vi "Lab Panel V4.82.vi"() -> ()   [LabVIEW 2013] (continued)
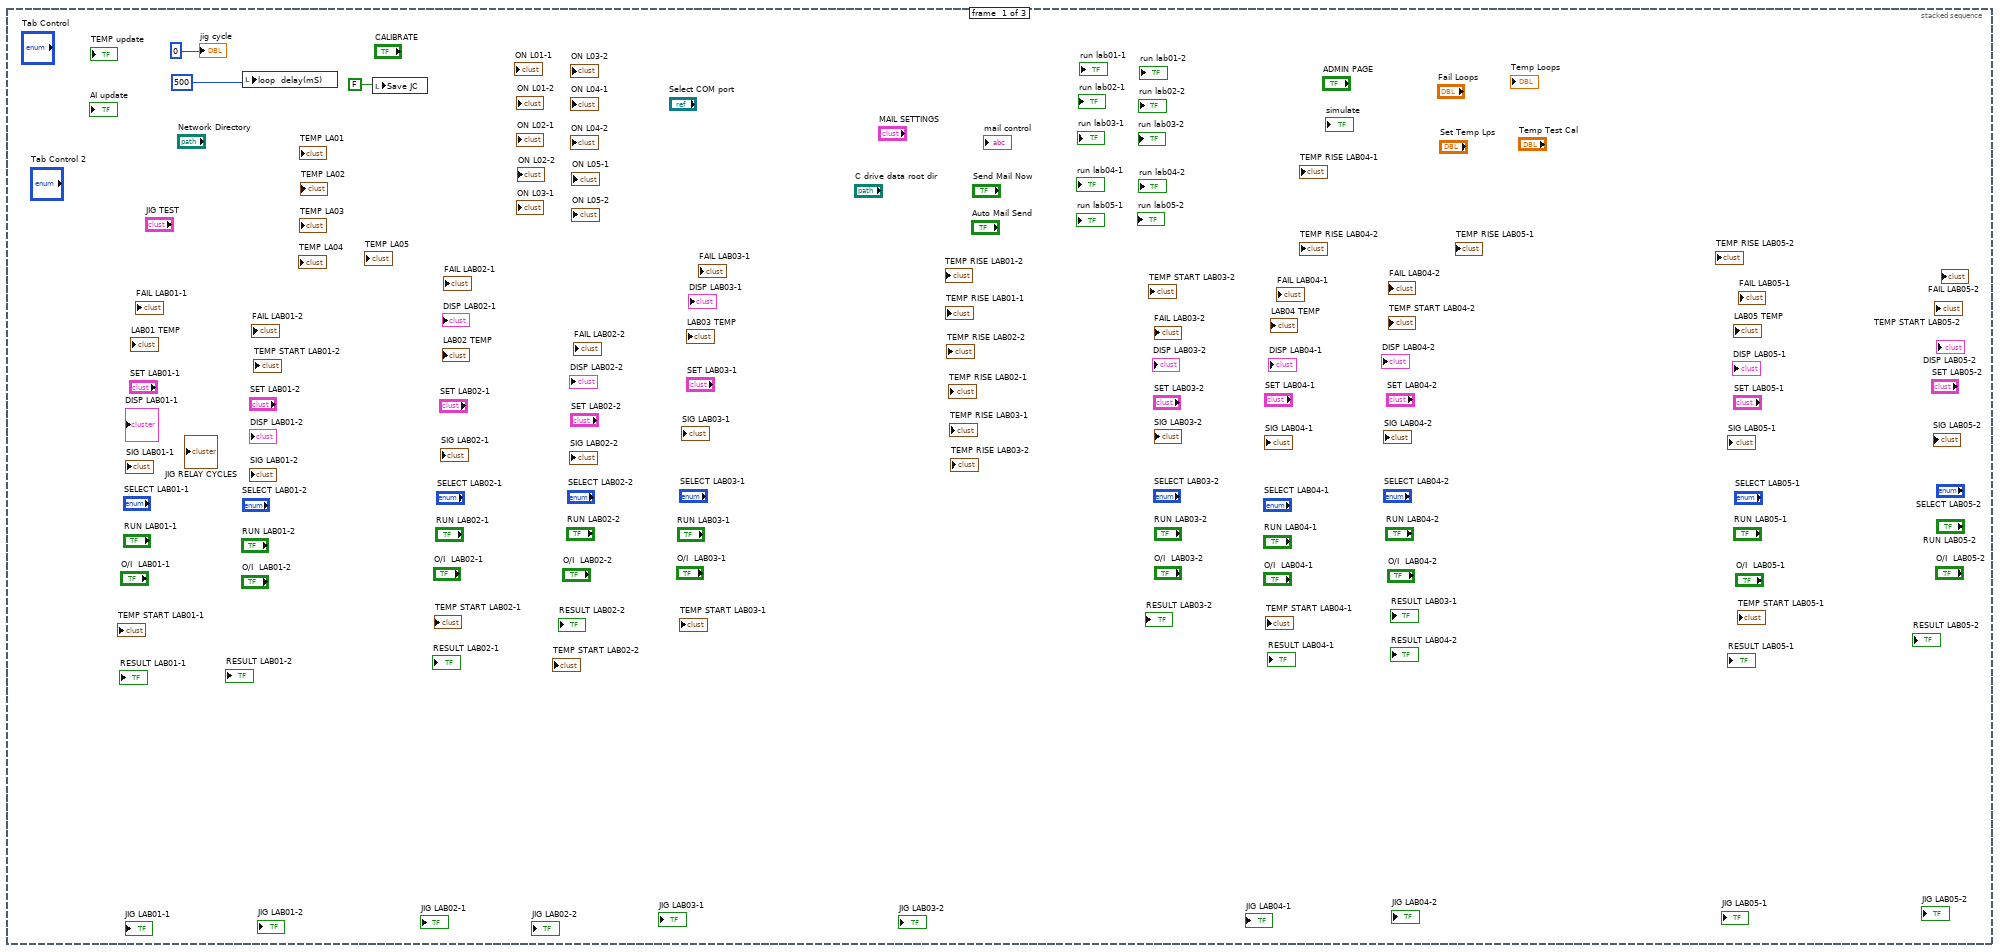
[diagram p2: hidden frame]
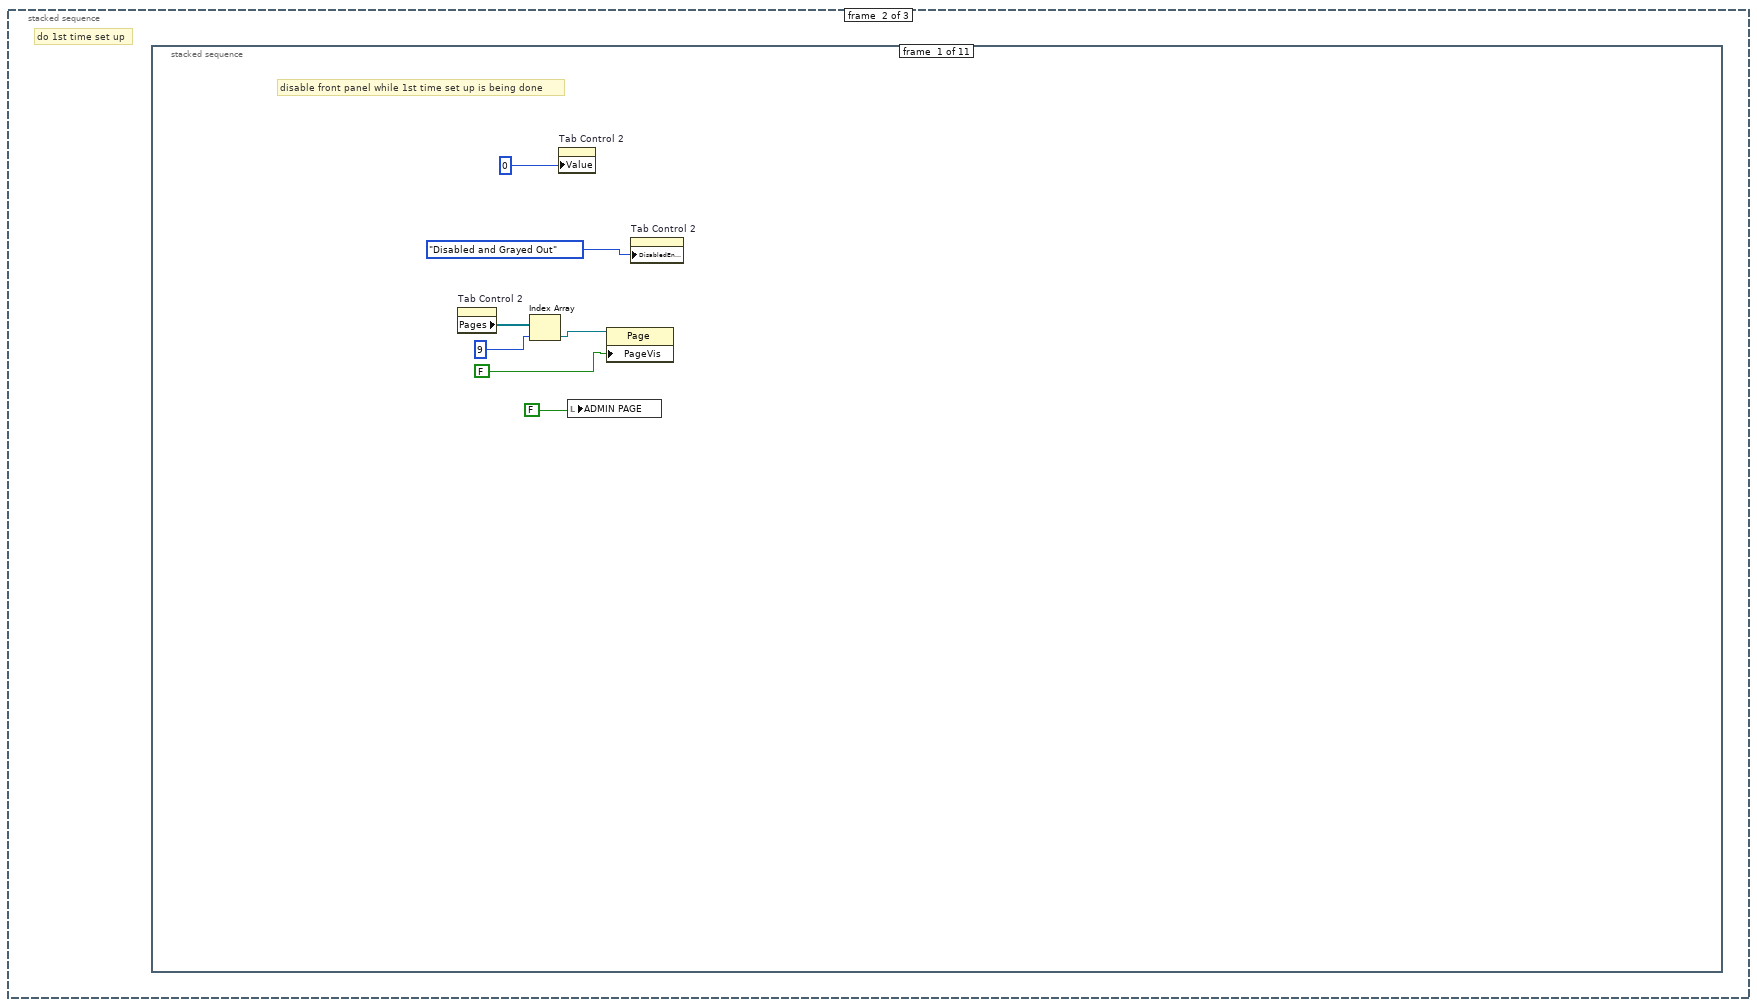
[diagram p3: hidden frame]
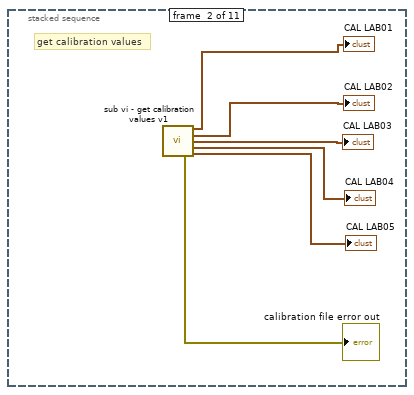
[diagram p4: hidden frame]
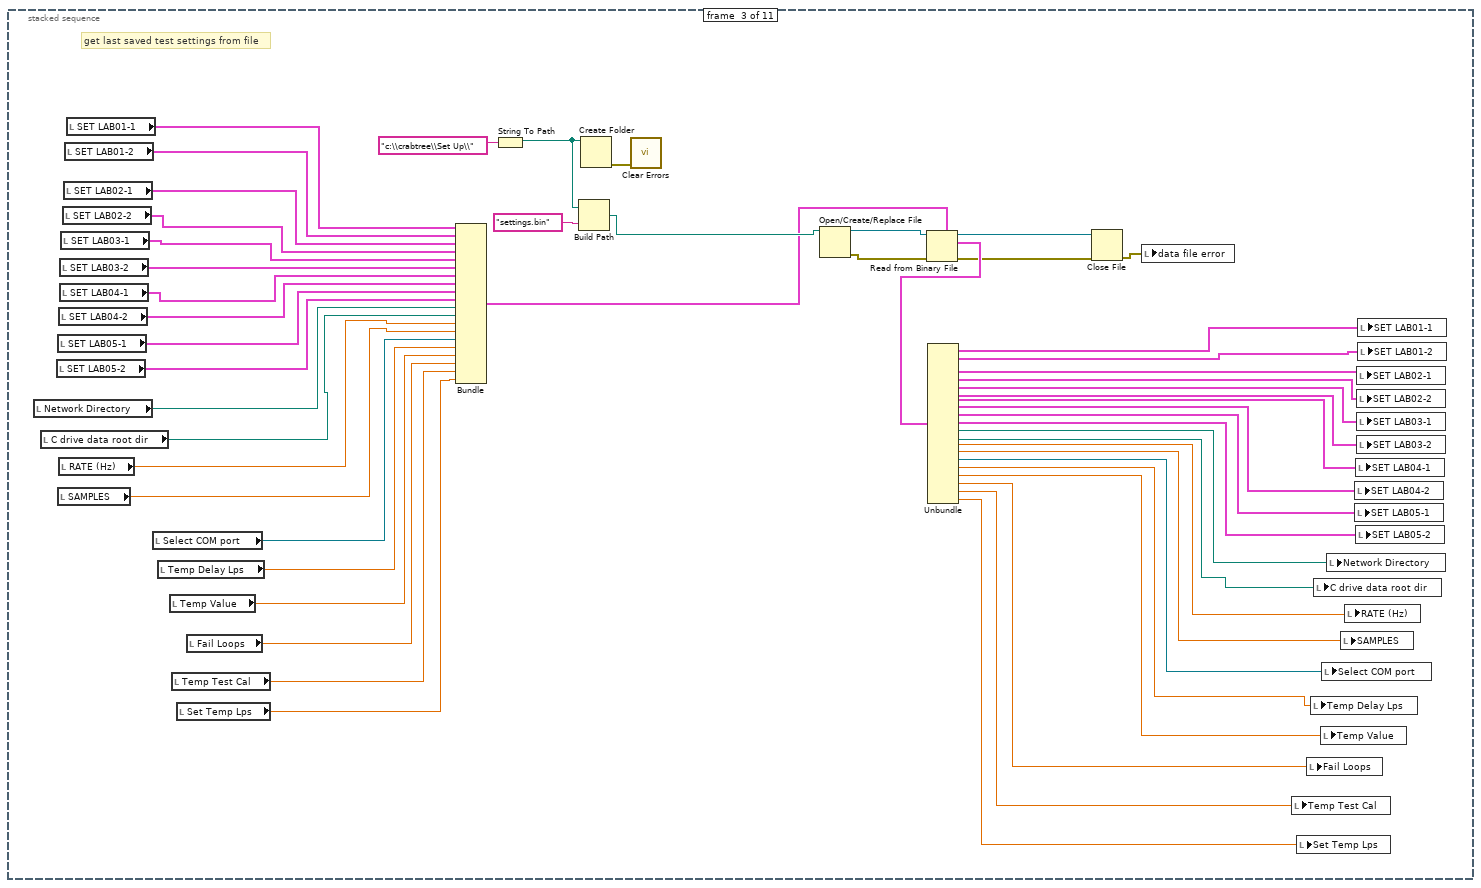
[diagram p5: hidden frame]
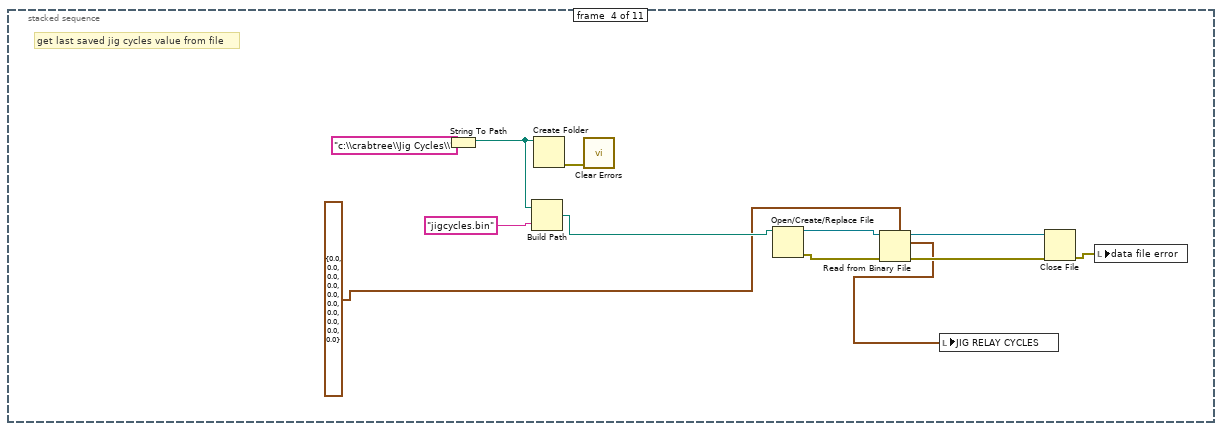
[diagram p6: hidden frame]
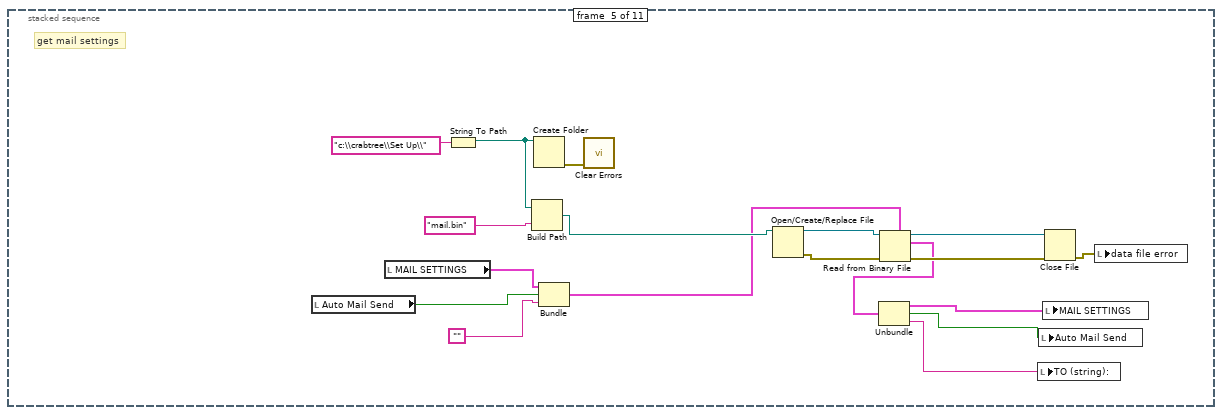
[diagram p7: hidden frame]
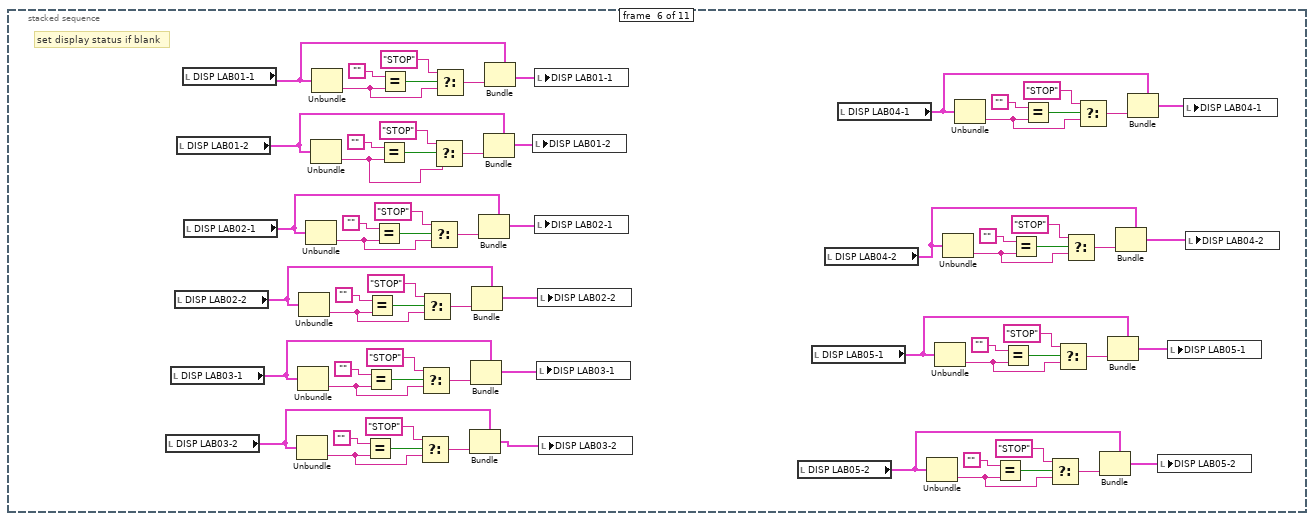
[diagram p8: hidden frame]
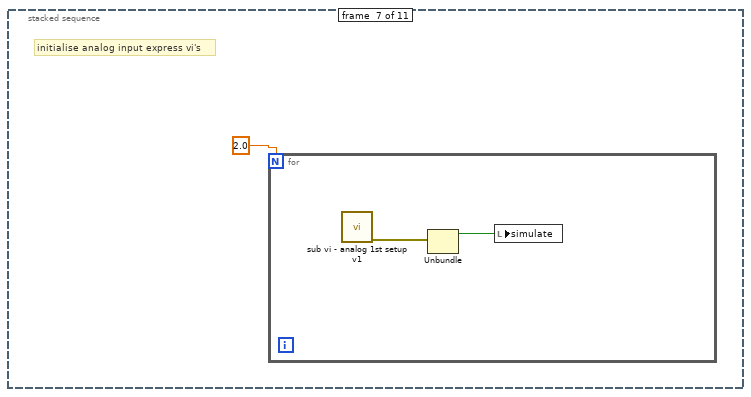
[diagram p9: hidden frame]
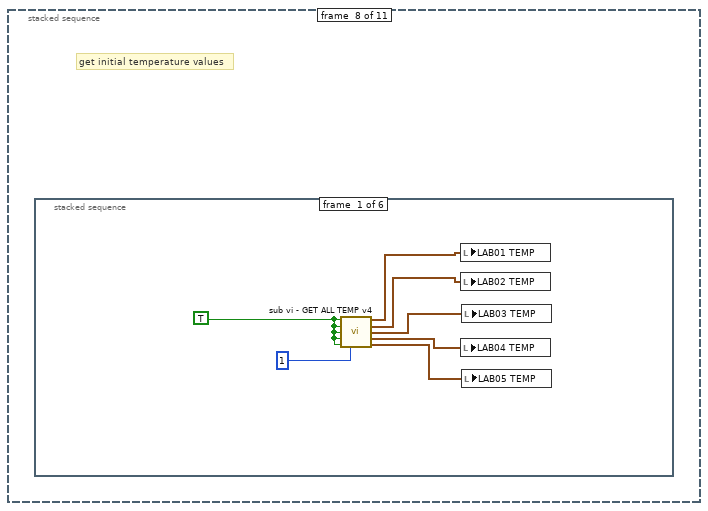
[diagram p10: hidden frame]
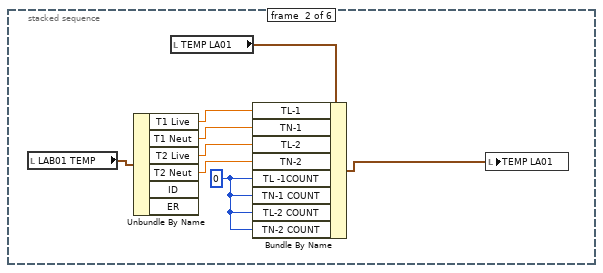
[diagram p11: hidden frame]
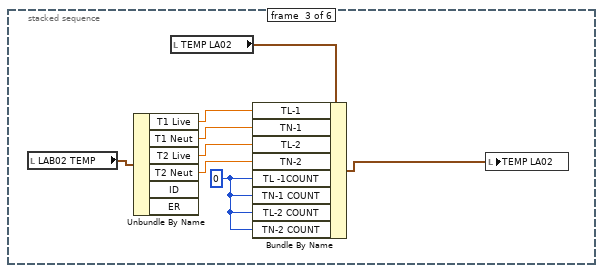
[diagram p12: hidden frame]
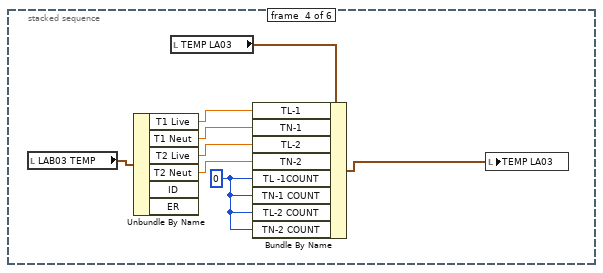
[diagram p13: hidden frame]
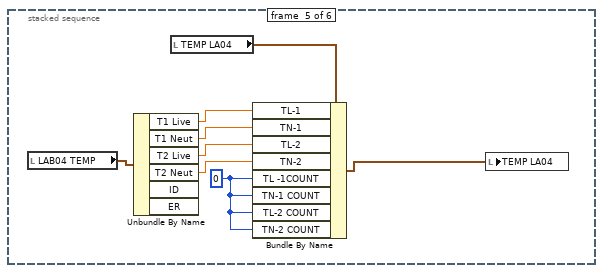
[diagram p14: hidden frame]
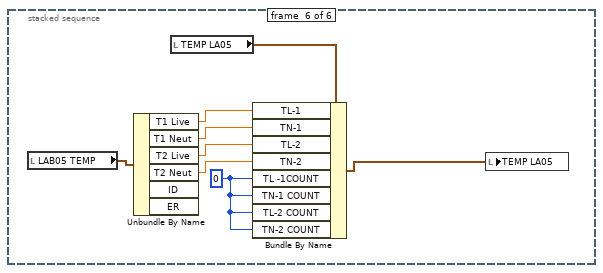
[diagram p15: hidden frame]
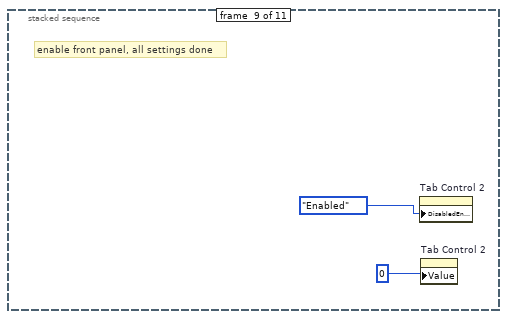
[diagram p16: hidden frame]
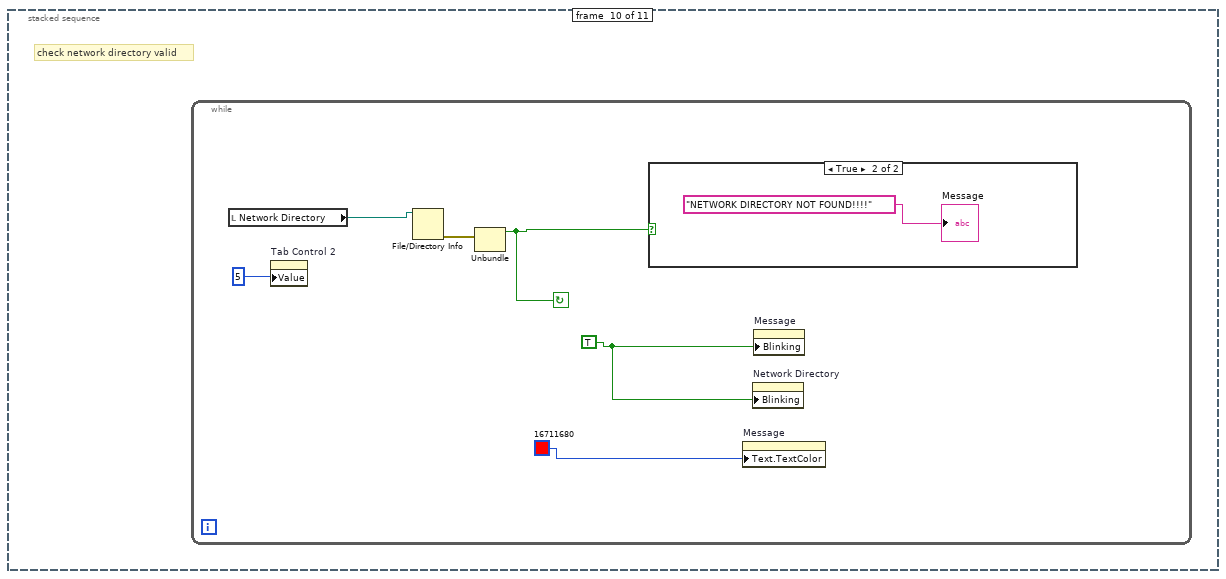
[diagram p17: hidden frame]
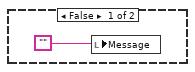
[diagram p18: hidden frame]
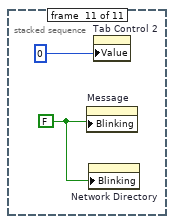
[diagram p19: hidden frame]
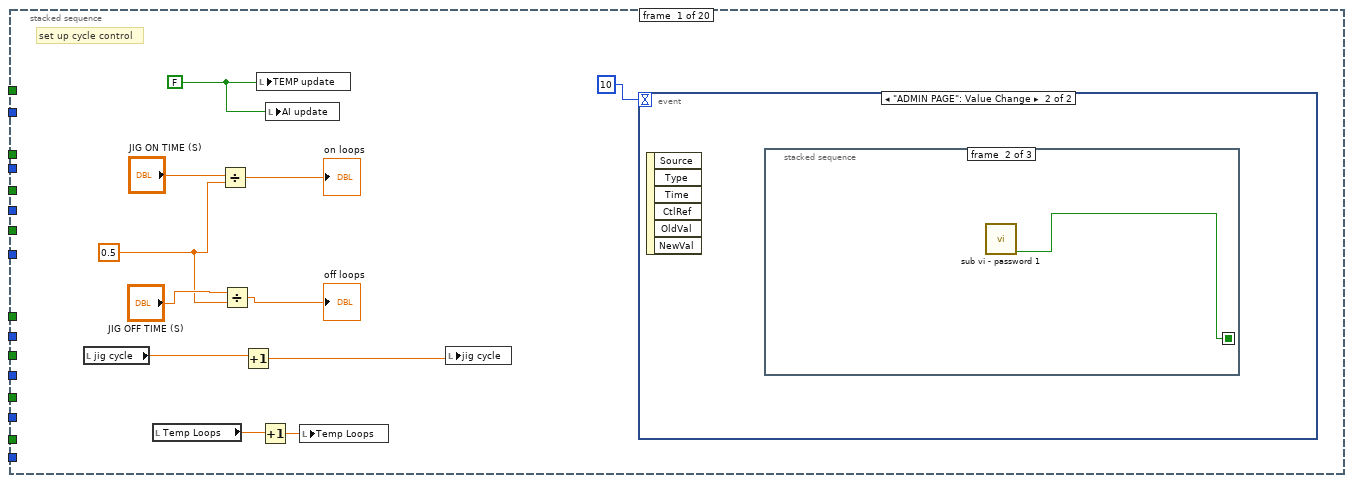
[diagram p20: hidden frame]
                            n2643 = Greater?(x=w4490, y=w4493) -> (0:w4492:bool)
                            n2644 = case shown="True" w4492 {
                              tunnel: [w4494 0] -> w4491
                              tunnel: w4490 -> [w4494 _]
                              tunnel: w4489 -> [_ w4495]
                              frame False {
                              }
                              frame True {
                                n2645 = Concatenate Strings("LA01-1 ", w4495) -> (w4498:string)
                                n2646 = One Button Dialog(message=w4498) -> ()  [unwired: 1 in, 1 out]
                              }
                            }
                          }
                          frame #1 {
                            n2647 = Greater?(x=w4499, y=w4503) -> (0:w4502:bool)
                            n2648 = case shown="True" w4502 {
                              tunnel: [w4504 0] -> w4500
                              tunnel: w4499 -> [w4504 _]
                              tunnel: w4501 -> [_ w4505]
                              frame False {
                              }
                              frame True {
                                n2649 = Concatenate Strings("LA01-2 ", w4505) -> (w4508:string)
                                n2650 = One Button Dialog(message=w4508) -> ()  [unwired: 1 in, 1 out]
                              }
                            }
                          }
                          frame #2 {
                            n2651 = Greater?(x=w4509, y=w4513) -> (0:w4512:bool)
                            n2652 = case shown="True" w4512 {
                              tunnel: [w4514 0] -> w4510
                              tunnel: w4509 -> [w4514 _]
                              tunnel: w4511 -> [_ w4515]
                              frame False {
                              }
                              frame True {
                                n2653 = Concatenate Strings("LA02-1 ", w4515) -> (w4518:string)
                                n2654 = One Button Dialog(message=w4518) -> ()  [unwired: 1 in, 1 out]
                              }
                            }
                          }
                          frame #3 {
                            n2655 = Greater?(x=w4520, y=w4523) -> (0:w4522:bool)
                            n2656 = case shown="True" w4522 {
                              tunnel: [w4524 0] -> w4519
                              tunnel: w4520 -> [w4524 _]
                              tunnel: w4521 -> [_ w4525]
                              frame False {
                              }
                              frame True {
                                n2657 = Concatenate Strings("LA02-2 ", w4525) -> (w4528:string)
                                n2658 = One Button Dialog(message=w4528) -> ()  [unwired: 1 in, 1 out]
                              }
                            }
                          }
                          frame #4 {
                            n2659 = Greater?(x=w4530, y=w4533) -> (0:w4532:bool)
                            n2660 = case shown="True" w4532 {
                              tunnel: [w4534 0] -> w4529
                              tunnel: w4530 -> [w4534 _]
                              tunnel: w4531 -> [_ w4535]
                              frame False {
                              }
                              frame True {
                                n2661 = Concatenate Strings("LA03-1 ", w4535) -> (w4538:string)
                                n2662 = One Button Dialog(message=w4538) -> ()  [unwired: 1 in, 1 out]
                              }
                            }
                          }
                          frame #5 {
                            n2663 = Greater?(x=w4539, y=w4543) -> (0:w4542:bool)
                            n2664 = case shown="True" w4542 {
                              tunnel: [w4544 0] -> w4540
                              tunnel: w4539 -> [w4544 _]
                              tunnel: w4541 -> [_ w4545]
                              frame False {
                              }
                              frame True {
                                n2665 = Concatenate Strings("LA03-2 ", w4545) -> (w4548:string)
                                n2666 = One Button Dialog(message=w4548) -> ()  [unwired: 1 in, 1 out]
                              }
                            }
                          }
                          frame #6 {
                            n2667 = Greater?(x=w4550, y=w4553) -> (0:w4552:bool)
                            n2668 = case shown="True" w4552 {
                              tunnel: [w4554 0] -> w4549
                              tunnel: w4550 -> [w4554 _]
                              tunnel: w4551 -> [_ w4555]
                              frame False {
                              }
                              frame True {
                                n2669 = Concatenate Strings("LA04-1 ", w4555) -> (w4558:string)
                                n2670 = One Button Dialog(message=w4558) -> ()  [unwired: 1 in, 1 out]
                              }
                            }
                          }
                          frame #7 {
                            n2671 = Greater?(x=w4560, y=w4563) -> (0:w4562:bool)
                            n2672 = case shown="True" w4562 {
                              tunnel: [w4564 0] -> w4559
                              tunnel: w4560 -> [w4564 _]
                              tunnel: w4561 -> [_ w4565]
                              frame False {
                              }
                              frame True {
                                n2673 = Concatenate Strings("LA04-2 ", w4565) -> (w4568:string)
                                n2674 = One Button Dialog(message=w4568) -> ()  [unwired: 1 in, 1 out]
                              }
                            }
                          }
                          frame #8 {
                            n2675 = Greater?(x=w4570, y=w4573) -> (0:w4572:bool)
                            n2676 = case shown="True" w4572 {
                              tunnel: [w4574 0] -> w4569
                              tunnel: w4570 -> [w4574 _]
                              tunnel: w4571 -> [_ w4575]
                              frame False {
                              }
                              frame True {
                                n2677 = Concatenate Strings("LA05-1 ", w4575) -> (w4578:string)
                                n2678 = One Button Dialog(message=w4578) -> ()  [unwired: 1 in, 1 out]
                              }
                            }
                          }
                          frame #9 {
                            n2679 = Greater?(x=w4580, y=w4583) -> (0:w4582:bool)
                            n2680 = case shown="True" w4582 {
                              tunnel: [w4584 0] -> w4579
                              tunnel: w4580 -> [w4584 _]
                              tunnel: w4581 -> [_ w4585]
                              frame False {
                              }
                              frame True {
                                n2681 = Concatenate Strings("LA05-2 ", w4585) -> (w4588:string)
                                n2682 = One Button Dialog(message=w4588) -> ()  [unwired: 1 in, 1 out]
                              }
                            }
                          }
                        }
                        n2683 = Bundle By Name(cluster=w4487, "LAB01-1"=w4485, "LAB01-2"=w4483, "LAB02-1"=w4480, "LAB02-2"=w4477, "LAB03-1"=w4475, "LAB03-2"=w4474, "LAB04-1"=w4471, "LAB04-2"=w4469, "LAB05-1"=w4467, "LAB05-2"=w4465) -> (w4486:T10)
                        n2684 = local write "JIG RELAY CYCLES"(w4486) -> ()
                      }
                    }
                  }
                }
              }
            }
          }
          frame #19 {
            # "get temperature values"
            n2685 = local read "simulate"() -> (w4593:bool)
            n2686 = local read "Temp Test Cal"() -> (w4590:dbl)
            n2687 = stacked-sequence {
              tunnel: w4593 -> [_ w4631 w4660 w4684 w4708 w4732]
              tunnel: T8 {"1  (A) cal"=1.0, "1 (V) cal"=1.0, "1 (PF) cal"=1.0, "1 (TL) cal"=1.0, "1 (TN) cal"=1.0, "2 (A) cal"=1.0, "2 (V) cal"=1.0, "2 (PF) cal"=1.0, "2 (TL) cal"=1.0, "2 (TN) cal"=1.0} ("CAL LAB01") -> [_ w4630 w4659 w4683 w4707 w4731]
              tunnel: w4591 -> [_ w4628 _ _ _ _]
              tunnel: w4590 -> [_ w4626 _ _ _ _]
              tunnel: w4589 -> [_ _ _ _ _ _]
              frame #0 {
                n2688 = local read "Select COM port"() -> (w4602:refnum<visa-resource-name>)
                "COM port" <- w4602
                n2689 = local read "Set Temp Lps"() -> (w4594:dbl)
                n2690 = local read "jig cycle"() -> (w4603:dbl)
                n2691 = local read "on loops"() -> (w4605:dbl)
                n2692 = local read "Temp Loops"() -> (w4598:dbl)
                n2693 = global write "Global 1.vi" "tmp dly lps"("Temp Delay Lps") -> ()
                n2694 = global write "Global 1.vi" "dly value"("Temp Value") -> ()
                n2695 = Add(x=w4605, y=3) -> (x+y=w4606:dbl)
                n2696 = global write "Global 1.vi" "COM port"(w4602) -> ()
                n2697 = Equal?(x=w4603, y=w4606) -> (x = y?=w4597:bool)
                n2698 = Greater Or Equal?(x=w4598, y=w4594) -> (x >= y?=w4596:bool)
                n2699 = And(x=w4597, y=w4596) -> (x .and. y?=w4595:bool)
                n2700 = local read "simulate"() -> (w4599:bool)
                n2701 = case shown="True" w4595 {
                  tunnel: w4599 -> [_ w4611]
                  frame False {
                  }
                  frame True {
                    n2702 = case shown="False" w4611 {
                      tunnel: [w4619 w4623] -> w4613
                      tunnel: [w4618 w4623] -> w4612
                      tunnel: [w4617 w4623] -> w4610
                      tunnel: [w4616 w4623] -> w4609
                      tunnel: [w4615 w4623] -> w4608
                      frame False {
                        w4621 = TRUE
                        w4622 = TRUE
                        n2703 = call "sub vi - GET ALL TEMP v4.vi"("LA01-EN"=w4622, "LA02-EN"=w4622, "LA03-EN"=w4622, "LA04-EN"=w4621, "LA05-EN"=w4621, "Gen Cal Value"=1.0) -> ("LA01 TEMP"=w4615:T23, "LA02 TEMP"=w4616:T23, "LA03 TEMP"=w4617:T23, "LA04 TEMP"=w4619:T23, "LA05 TEMP"=w4618:T23)  [unwired: 4 in, 1 out]
                      }
                      frame True {
                        w4623 = T14 {"T1 Live"=21.0, "T1 Neut"=22.0, "T2 Live"=23.0, "T2 Neut"=24.0, "ID"=6.0, "ER"=10.0} ("LAB01 TEMP")
                      }
                    }
                    n2704 = local write "Temp Loops"(0) -> ()
                    n2705 = local write "TEMP update"(TRUE) -> ()
                    n2706 = local write "LAB03 TEMP"(w4610) -> ()
                    n2707 = local write "LAB02 TEMP"(w4609) -> ()
                    n2708 = local write "LAB04 TEMP"(w4613) -> ()
                    n2709 = local write "LAB05 TEMP"(w4612) -> ()
                    n2710 = local write "LAB01 TEMP"(w4608) -> ()
                  }
                }
              }
              frame #1 {
                n2711 = case shown="False" w4631 {
                  tunnel: [w4657 w4658] -> w4649
                  tunnel: w4630 -> [_ w4658]
                  frame False {
                    n2712 = local read "CAL LAB01"() -> (w4657:T8)
                  }
                  frame True {
                  }
                }
                n2713 = local read "LAB01 TEMP"() -> (w4637:T14)
                n2714 = local read "TEMP LA01"() -> (w4638:T11)
                n2715 = call "sub vi - temperature delay v2.vi"("temp values IN"=w4638, "temp signals"=w4637) -> ("T2-N"=w4633:dbl, "T2-L"=w4634:dbl, "T1-N"=w4635:dbl, "T1-L"=w4636:dbl, "temp values OUT"=w4632:T43)  [unwired: 5 in]
                n2716 = Unbundle By Name(w4649) -> ("1 (TL) cal"=w4642:dbl, "1 (TN) cal"=w4641:dbl, "2 (TL) cal"=w4640:dbl, "2 (TN) cal"=w4639:dbl)  [unwired: 6 out]
                n2717 = local write "TEMP LA01"(w4632) -> ()
                n2718 = Multiply(x=w4636, y=w4642) -> (x*y=w4629:dbl)
                n2719 = Multiply(x=w4635, y=w4641) -> (x*y=w4625:dbl)
                n2720 = Multiply(x=w4634, y=w4640) -> (x*y=w4644:dbl)
                n2721 = Multiply(x=w4633, y=w4639) -> (x*y=w4643:dbl)
                n2722 = case shown="True" w4628 {
                  tunnel: w4629 -> [w4651 w4656]
                  tunnel: w4626 -> [_ w4654]
                  tunnel: [w4651 w4655] -> w4627
                  tunnel: w4625 -> [w4650 w4653]
                  tunnel: [w4650 w4652] -> w4624
                  frame False {
                  }
                  frame True {
                    n2723 = Multiply(x=w4654, y=w4653) -> (x*y=w4652:dbl)
                    n2724 = Multiply(x=w4654, y=w4656) -> (x*y=w4655:dbl)
                  }
                }
                n2725 = local read "SIG LAB01-2"() -> (w4646:T2)
                n2726 = local read "SIG LAB01-1"() -> (w4648:T2)
                n2727 = Bundle By Name(cluster=w4648, "Tmp Live"=w4627, "Tmp Neut"=w4624) -> (w4647:T2)
                n2728 = Bundle By Name(cluster=w4646, "Tmp Live"=w4644, "Tmp Neut"=w4643) -> (w4645:T2)
                n2729 = local write "SIG LAB01-1"(w4647) -> ()
                n2730 = local write "SIG LAB01-2"(w4645) -> ()
              }
              frame #2 {
                n2731 = case shown="True" w4660 {
                  tunnel: [w4681 w4682] -> w4680
                  tunnel: w4659 -> [_ w4682]
                  frame False {
                    n2732 = local read "CAL LAB02"() -> (w4681:T9)
                  }
                  frame True {
                  }
                }
                n2733 = local read "LAB02 TEMP"() -> (w4667:T14)
                n2734 = local read "TEMP LA02"() -> (w4666:T11)
                n2735 = call "sub vi - temperature delay v2.vi"("temp values IN"=w4666, "temp signals"=w4667) -> ("T2-N"=w4661:dbl, "T2-L"=w4662:dbl, "T1-N"=w4663:dbl, "T1-L"=w4664:dbl, "temp values OUT"=w4665:T43)  [unwired: 5 in]
                n2736 = Unbundle By Name(w4680) -> ("1 (TL) cal"=w4671:dbl, "1 (TN) cal"=w4670:dbl, "2 (TL) cal"=w4669:dbl, "2 (TN) cal"=w4668:dbl)  [unwired: 6 out]
                n2737 = local write "TEMP LA02"(w4665) -> ()
                n2738 = Multiply(x=w4664, y=w4671) -> (x*y=w4677:dbl)
                n2739 = Multiply(x=w4663, y=w4670) -> (x*y=w4676:dbl)
                n2740 = Multiply(x=w4662, y=w4669) -> (x*y=w4673:dbl)
                n2741 = Multiply(x=w4661, y=w4668) -> (x*y=w4672:dbl)
                n2742 = local read "SIG LAB02-2"() -> (w4675:T2)
                n2743 = local read "SIG LAB02-1"() -> (w4679:T2)
                n2744 = Bundle By Name(cluster=w4679, "Tmp Live"=w4677, "Tmp Neut"=w4676) -> (w4678:T2)
                n2745 = Bundle By Name(cluster=w4675, "Tmp Live"=w4673, "Tmp Neut"=w4672) -> (w4674:T2)
                n2746 = local write "SIG LAB02-1"(w4678) -> ()
                n2747 = local write "SIG LAB02-2"(w4674) -> ()
              }
              frame #3 {
                n2748 = case shown="False" w4684 {
                  tunnel: [w4705 w4706] -> w4704
                  tunnel: w4683 -> [_ w4706]
                  frame False {
                    n2749 = local read "CAL LAB03"() -> (w4705:T8)
                  }
                  frame True {
                  }
                }
                n2750 = local read "TEMP LA03"() -> (w4690:T11)
                n2751 = local read "LAB03 TEMP"() -> (w4691:T14)
                n2752 = call "sub vi - temperature delay v2.vi"("temp values IN"=w4690, "temp signals"=w4691) -> ("T2-N"=w4685:dbl, "T2-L"=w4686:dbl, "T1-N"=w4687:dbl, "T1-L"=w4688:dbl, "temp values OUT"=w4689:T43)  [unwired: 5 in]
                n2753 = Unbundle By Name(w4704) -> ("1 (TL) cal"=w4695:dbl, "1 (TN) cal"=w4694:dbl, "2 (TL) cal"=w4693:dbl, "2 (TN) cal"=w4692:dbl)  [unwired: 6 out]
                n2754 = local write "TEMP LA03"(w4689) -> ()
                n2755 = Multiply(x=w4688, y=w4695) -> (x*y=w4701:dbl)
                n2756 = Multiply(x=w4687, y=w4694) -> (x*y=w4700:dbl)
                n2757 = Multiply(x=w4686, y=w4693) -> (x*y=w4697:dbl)
                n2758 = Multiply(x=w4685, y=w4692) -> (x*y=w4696:dbl)
                n2759 = local read "SIG LAB03-2"() -> (w4699:T2)
                n2760 = local read "SIG LAB03-1"() -> (w4703:T2)
                n2761 = Bundle By Name(cluster=w4703, "Tmp Live"=w4701, "Tmp Neut"=w4700) -> (w4702:T2)
                n2762 = Bundle By Name(cluster=w4699, "Tmp Live"=w4697, "Tmp Neut"=w4696) -> (w4698:T2)
                n2763 = local write "SIG LAB03-1"(w4702) -> ()
                n2764 = local write "SIG LAB03-2"(w4698) -> ()
              }
              frame #4 {
                n2765 = case shown="False" w4708 {
                  tunnel: [w4729 w4730] -> w4728
                  tunnel: w4707 -> [_ w4730]
                  frame False {
                    n2766 = local read "CAL LAB04"() -> (w4729:T8)
                  }
                  frame True {
                  }
                }
                n2767 = local read "LAB04 TEMP"() -> (w4714:T14)
                n2768 = local read "TEMP LA04"() -> (w4715:T11)
                n2769 = call "sub vi - temperature delay v2.vi"("temp values IN"=w4715, "temp signals"=w4714) -> ("T2-N"=w4709:dbl, "T2-L"=w4710:dbl, "T1-N"=w4711:dbl, "T1-L"=w4712:dbl, "temp values OUT"=w4713:T43)  [unwired: 5 in]
                n2770 = Unbundle By Name(w4728) -> ("1 (TL) cal"=w4719:dbl, "1 (TN) cal"=w4718:dbl, "2 (TL) cal"=w4717:dbl, "2 (TN) cal"=w4716:dbl)  [unwired: 6 out]
                n2771 = local write "TEMP LA04"(w4713) -> ()
                n2772 = Multiply(x=w4712, y=w4719) -> (x*y=w4725:dbl)
                n2773 = Multiply(x=w4711, y=w4718) -> (x*y=w4724:dbl)
                n2774 = Multiply(x=w4710, y=w4717) -> (x*y=w4721:dbl)
                n2775 = Multiply(x=w4709, y=w4716) -> (x*y=w4720:dbl)
                n2776 = local read "SIG LAB04-2"() -> (w4723:T2)
                n2777 = local read "SIG LAB04-1"() -> (w4727:T2)
                n2778 = Bundle By Name(cluster=w4727, "Tmp Live"=w4725, "Tmp Neut"=w4724) -> (w4726:T2)
                n2779 = Bundle By Name(cluster=w4723, "Tmp Live"=w4721, "Tmp Neut"=w4720) -> (w4722:T2)
                n2780 = local write "SIG LAB04-1"(w4726) -> ()
                n2781 = local write "SIG LAB04-2"(w4722) -> ()
              }
              frame #5 {
                n2782 = case shown="False" w4732 {
                  tunnel: [w4753 w4754] -> w4752
                  tunnel: w4731 -> [_ w4754]
                  frame False {
                    n2783 = local read "CAL LAB05"() -> (w4753:T8)
                  }
                  frame True {
                  }
                }
                n2784 = local read "LAB05 TEMP"() -> (w4738:T14)
                n2785 = local read "TEMP LA05"() -> (w4739:T11)
                n2786 = call "sub vi - temperature delay v2.vi"("temp values IN"=w4739, "temp signals"=w4738) -> ("T2-N"=w4734:dbl, "T2-L"=w4735:dbl, "T1-N"=w4736:dbl, "T1-L"=w4737:dbl, "temp values OUT"=w4733:T43)  [unwired: 5 in]
                n2787 = local write "TEMP LA05"(w4733) -> ()
                n2788 = Unbundle By Name(w4752) -> ("1 (TL) cal"=w4740:dbl, "1 (TN) cal"=w4743:dbl, "2 (TL) cal"=w4742:dbl, "2 (TN) cal"=w4741:dbl)  [unwired: 6 out]
                n2789 = Multiply(x=w4737, y=w4740) -> (x*y=w4749:dbl)
                n2790 = Multiply(x=w4736, y=w4743) -> (x*y=w4748:dbl)
                n2791 = Multiply(x=w4735, y=w4742) -> (x*y=w4745:dbl)
                n2792 = Multiply(x=w4734, y=w4741) -> (x*y=w4744:dbl)
                n2793 = local read "SIG LAB05-2"() -> (w4747:T2)
                n2794 = local read "SIG LAB05-1"() -> (w4751:T2)
                n2795 = Bundle By Name(cluster=w4751, "Tmp Live"=w4749, "Tmp Neut"=w4748) -> (w4750:T2)
                n2796 = Bundle By Name(cluster=w4747, "Tmp Live"=w4745, "Tmp Neut"=w4744) -> (w4746:T2)
                n2797 = local write "SIG LAB05-1"(w4750) -> ()
                n2798 = local write "SIG LAB05-2"(w4746) -> ()
              }
            }
          }
        }
        n2799 = node-c288() -> ()  [unwired: 1 in, 1 out]
        "loops" <- w255
      }
      n2800 = node-c288(w232) -> ()  [unwired: 1 out]
    }
  }
